vi "Window_waveform.vi"(10 "beta in":dbl, 11 "waveform in":waveform(dbl)) -> (3 "Waveform":waveform(dbl))   [LabVIEW 2015]
uses:
  <vilib>/Analysis/4window.llb/Kaiser-Bessel Window (DBL).vi
  <vilib>/Analysis/NI_AALPro.lvlib
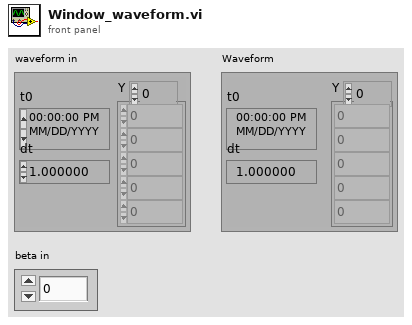
[diagram p1: front panel]
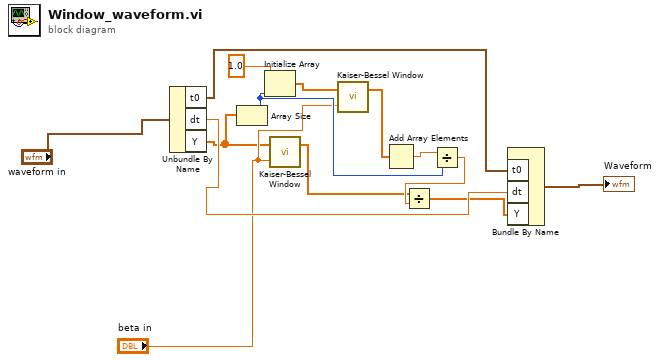
[diagram p0: block diagram]
diagram:
  n1 = Unbundle By Name("waveform in") -> ("t0"=w12:timestamp, "dt"=w13:dbl, "Y"=w3:dbl[])
  n2 = Array Size(array=w3) -> (size(s)=w9:i32)
  n3 = Initialize Array(1.0 ("element"), w9) -> (w4:dbl[])
  n4 = call-poly <vilib>:"Kaiser-Bessel Window.vi"("beta"="beta in", "X"=w3) -> ("Windowed X"=w7:dbl[])  [unwired: 1 out]
  n5 = call-poly <vilib>:"Kaiser-Bessel Window.vi"("beta"="beta in", "X"=w4) -> ("Windowed X"=w6:dbl[])  [unwired: 1 out]
  n6 = Add Array Elements(numeric array=w6) -> (sum=w8:dbl)
  n7 = Divide(x=w8, y=w9) -> (x/y=w10:dbl)
  n8 = Divide(x=w7, y=w10) -> (x/y=w11:dbl[])
  n9 = Bundle By Name("t0"=w12, "dt"=w13, "Y"=w11) -> (→"Waveform":waveform(dbl))  [unwired: 1 in]
